vi "Initialize Attributes Core.vi"(8 "error in (no error)":errorcluster, 10 "Attribute Data":variant, 11 "BNT_ULx-MCSV-I in":refnum<class "BNT_ULx-MCSV-I.lvclass">) -> (0 "error out":errorcluster, 2 "MandatoryParameters":cluster{"Parameter":string, "found?":bool}[](array[cluster]), 3 "BNT_ULx-MCSV-I out":refnum<class "BNT_ULx-MCSV-I.lvclass">)   [LabVIEW 2021, in "BNT_ULx.lvlib" / "BNT_ULx-MCSV-I.lvclass"]
doc: "Initialize object attribute.\n\nUnique resources should be allocated elsewhere!"
uses:
  BNT_ULx-MCSV-I.lvclass
  BNT_ULx-MCSV-I.lvclass/BNT_ULx-MCSV-I.ctl
  BNT_ULx-MCSV/BNT_ULx-MCSV.lvclass
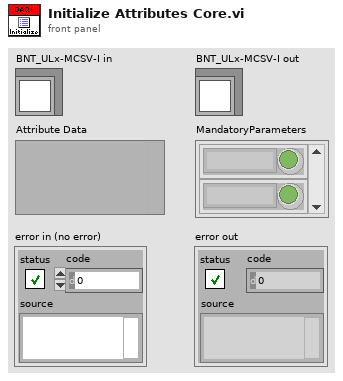
[diagram p1: front panel]
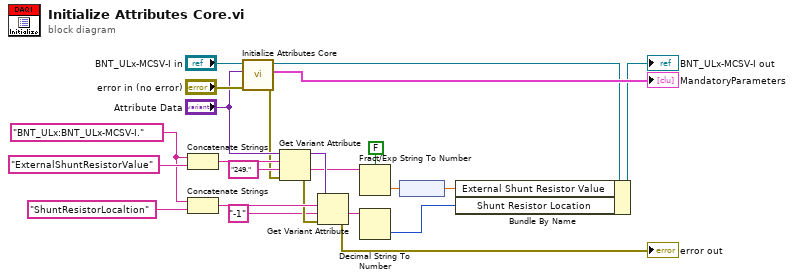
[diagram p0: block diagram]
diagram:
  w14 = "BNT_ULx:BNT_ULx-MCSV-I."
  n1 = Concatenate Strings(w14, "ExternalShuntResistorValue" ("string")) -> (w17:string)
  n2 = Concatenate Strings(w14, "ShuntResistorLocaltion" ("string")) -> (w19:string)
  n3 = call-parent "Initialize Attributes Core.vi"("error in (no error)"="error in (no error)", "Attribute Data"="Attribute Data", "BNT_ULx-MCSV in"="BNT_ULx-MCSV-I in") -> ("error out"=w3:errorcluster, "MandatoryParameters"=→"MandatoryParameters":cluster{"Parameter":string, "found?":bool}[], "BNT_ULx-MCSV out"=w9:refnum<class "BNT_ULx-MCSV-I.lvclass">)  [unwired: 6 in]
  n4 = Get Variant Attribute(Variant="Attribute Data", name=w17, default value (empty Variant)="249.", error in=w3) -> (duplicate Variant=w16:variant, value=w13:string, error out=w15:errorcluster)  [unwired: 1 out]
  n5 = Get Variant Attribute(Variant=w16, name=w19, default value (empty Variant)="-1", error in=w15) -> (value=w5:string, error out=→"error out":errorcluster)  [unwired: 2 out]
  n6 = Fract/Exp String To Number(use system decimal point (T)=FALSE, string=w13) -> (number=w11:dbl)  [unwired: 2 in, 1 out]
  n7 = Decimal String To Number(string=w5) -> (number=w4:i32)  [unwired: 2 in, 1 out]
  n8 = node(w11) -> (w6:dbl[unit])
  n9 = Bundle By Name(cluster=w9, "External Shunt Resistor Value"=w6, "Shunt Resistor Location"=w4) -> (→"BNT_ULx-MCSV-I out":refnum<class "BNT_ULx-MCSV-I.lvclass">)
